vi "Revision Query.vi"(8 "error in (no error)":errorcluster, 11 "VISA resource name":refnum<visa-resource-name>) -> (0 "error out":errorcluster, 1 "Firmware Revision":string, 2 "Instrument Driver Revision":string, 3 "VISA resource name out":refnum<visa-resource-name>)   [LabVIEW 2020, in "Rohde&Schwarz CMXP GPRF.lvlib"]
doc: "This VI returns the revision numbers of the instrument driver and instrument firmware.\n\nAttribute:\n-\n\nRemote-control command:\n*IDN?"
uses:
  <instrlib>/Rohde&Schwarz CMXP GPRF/Rohde&Schwarz CMXP GPRF.lvlib
  <instrlib>/Rohde&Schwarz CMXP GPRF/Private/rsidr_core.llb/rsidr_core.lvlib
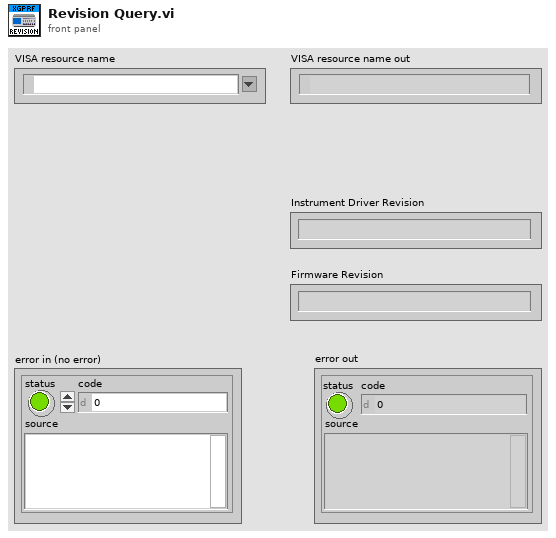
[diagram p1: front panel]
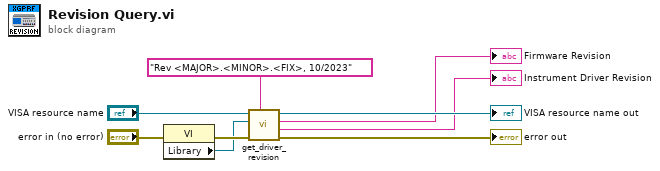
[diagram p0: block diagram]
diagram:
  n1 = property on="Property Node" class="VI"(error in="error in (no error)") -> (error out=w8:errorcluster, "Library"=w4:refnum<vi>)  [unwired: 1 in, 1 out]
  n2 = call <instrlib>:"get_driver_revision.vi"("Driver Version Formatting String"="Rev <MAJOR>.<MINOR>.<FIX>, 10/2023", "error in"=w8, "Library"=w4, "VISA resource name"="VISA resource name") -> ("error out"=→"error out":errorcluster, "Driver Version"=→"Instrument Driver Revision":string, "Instrument FW"=→"Firmware Revision":string, "VISA resource name out"=→"VISA resource name out":refnum<visa-resource-name>)  [unwired: 4 in]
